vi "Execute.vi"(5 "SleepTerminalArray":refnum<vi>, 6 "ExeRef":refnum<vi>, 7 "ActiveTerminalArray":refnum<vi>, 8 "error in (no error)":errorcluster, 9 "Json_In":string, 10 "VariableRef":T2, 11 "Info":T1) -> (0 "Error Out":errorcluster, 1 "NumResultArray":dbl[](array[numeric]), 2 "StrResultArray":string[](array[string]), 3 "StrResult":string, 4 "NumResult":dbl)   [LabVIEW 2018, in "File.lvlib"]
uses:
  File.lvlib
  <userlib>/_OpenG.lib/dictionary/dictionary.llb/Dictionary Object RefNum__ogtk.ctl
  <userlib>/_OpenG.lib/dictionary/dictionary.llb/Dictionary Object RefNum - Enum__ogtk.ctl
  <userlib>/_MGI/File/MGI Create Directory Chain Behavior Enum.ctl
  <vilib>/addons/_JKI.lib/Serialization/JSON/JKI JSON Serialization.lvlib
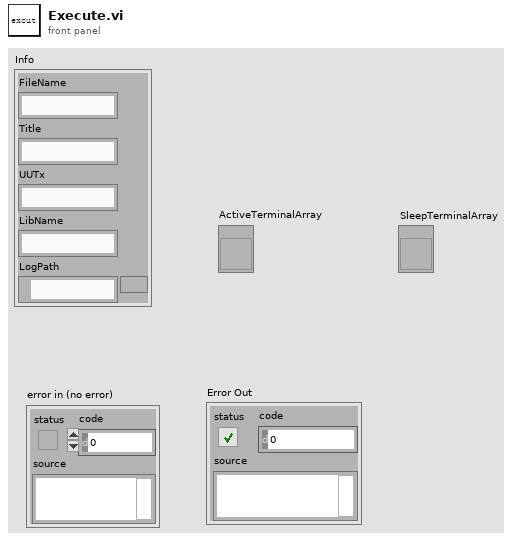
[diagram p1: front panel]
types:
  T1 = cluster{"FileName":string, "Title":string, "UUTx":string, "LibName":string, "LogPath":path}
  T2 = typedef "Dictionary Object RefNum__ogtk.ctl" = refnum<k1>
  T3 = cluster{"SetPath":cluster{"json":cluster{"Method":string, "Path":string, "PathType":string}}, "CreatFile":cluster{"json":cluster{"Method":string, "Path":string, "Operation":string, "Access":string, "DisableBuffering":bool}}, "CreatFolder":cluster{"json":cluster{"Method":string, "Path":string}}, "Delete":cluster{"json":cluster{"Method":string, "Path":string, "EntireHierarchy":bool, "Confirm":bool}}, "ReadTextFile":cluster{"json":cluster{"Method":string, "Path":string, "count":i32}}, "WriteTextFile":cluster{"json":cluster{"Method":string, "Path":string, "Offset":i64, "Position":string, "Text":string}}, "ReadBinFile":cluster{"json":cluster{"Method":string, "Path":string, "Count":i32, "ByteOrder":string}}, "WriteBinFile":cluster{"json":cluster{"Method":string, "Path":string, "ByteOrder":string, "PrependDataSize":bool, "Bin":string}}, "ReadFileMD5":cluster{"json":cluster{"Method":string, "Path":string}}, "Move":cluster{"json":cluster{"Method":string, "Path":string, "TargetPath":string, "Overwrite":bool}}, "Copy":cluster{"json":cluster{"Method":string, "Path":string, "TargetPath":string, "Overwrite":bool}}, "GetFileSize":cluster{"json":cluster{"Method":string, "Path":string}}, "CheckifFileorFolderExists":cluster{"json":cluster{"Method":string, "Path":string}}, "ListFolder":cluster{"json":cluster{"Method":string, "Path":string, "Type":string}}}
  T4 = typedef "MGI Create Directory Chain Behavior Enum.ctl" = enum16{"Auto Detect", "Path Contains a File", "Path Does Not Contain a File"}
  T5 = enum16{"open", "replace", "create", "open or create", "replace or create", "replace or create with confirmation"}
  T6 = enum16{"big-endian, network order", "native, host order", "little-endian"}
  T7 = cluster{"json":cluster{"Method":string, "Path":string, "PathType":string}}
  T8 = enum32{"invalid app kind", "Development System", "Run Time System", "Student Edition", "Embedded LabVIEW", "Evaluation", "Custom"}
  T9 = cluster{"json":cluster{"Method":string, "Path":string, "Operation":string, "Access":string, "DisableBuffering":bool}}
  T10 = cluster{"json":cluster{"Method":string, "Path":string}}
  T11 = cluster{"json":cluster{"Method":string, "Path":string, "EntireHierarchy":bool, "Confirm":bool}}
  T12 = cluster{"json":cluster{"Method":string, "Path":string, "count":i32}}
  T13 = cluster{"json":cluster{"Method":string, "Path":string, "Offset":i64, "Position":string, "Text":string}}
  T14 = cluster{"json":cluster{"Method":string, "Path":string, "Count":i32, "ByteOrder":string}}
  T15 = cluster{"json":cluster{"Method":string, "Path":string, "ByteOrder":string, "PrependDataSize":bool, "Bin":string}}
  T16 = cluster{"json":cluster{"Method":string, "Path":string, "TargetPath":string, "Overwrite":bool}}
  T17 = cluster{"json":cluster{"Method":string, "Path":string, "Type":string}}
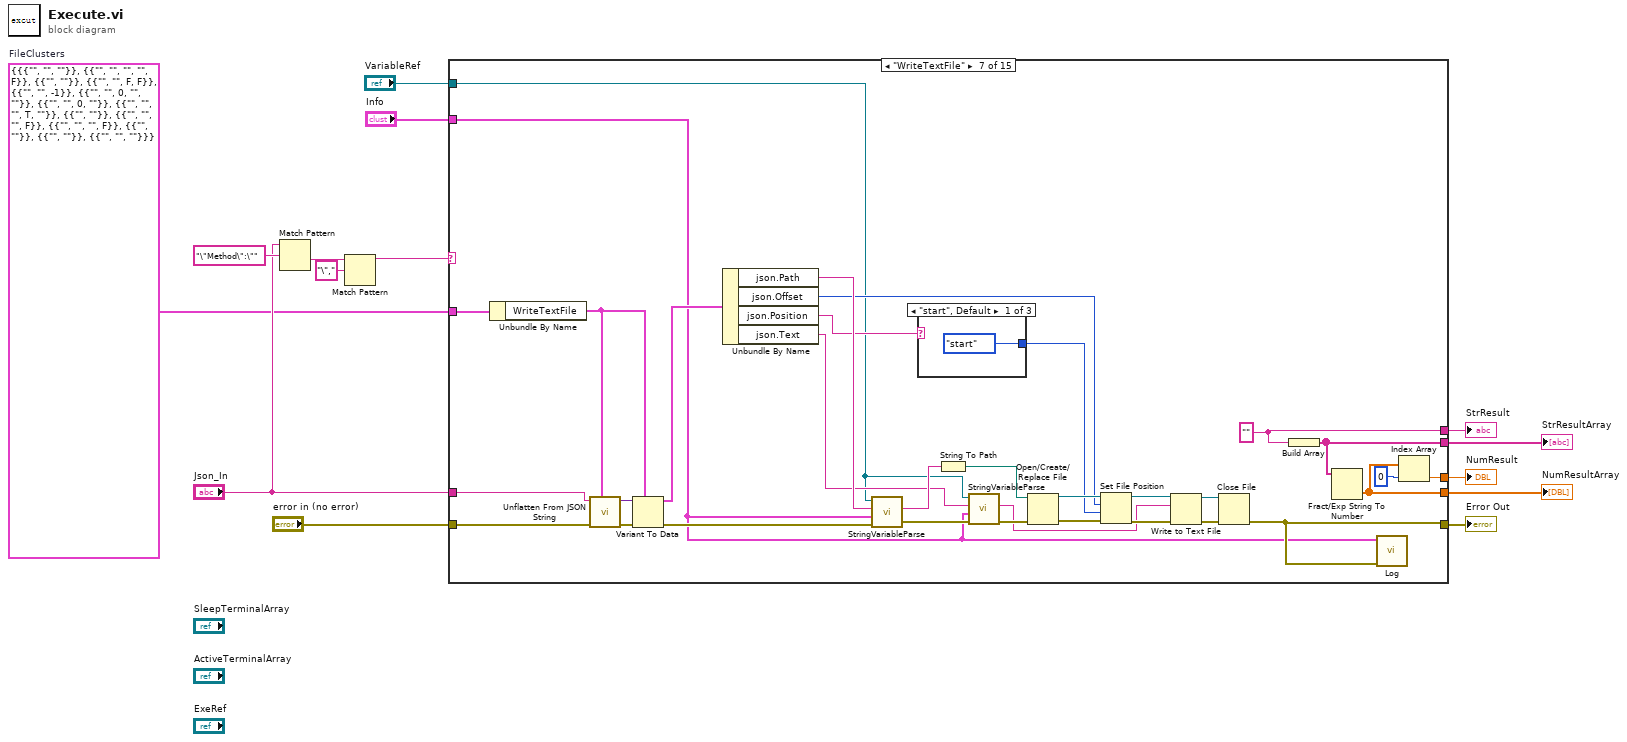
[diagram p0: block diagram]
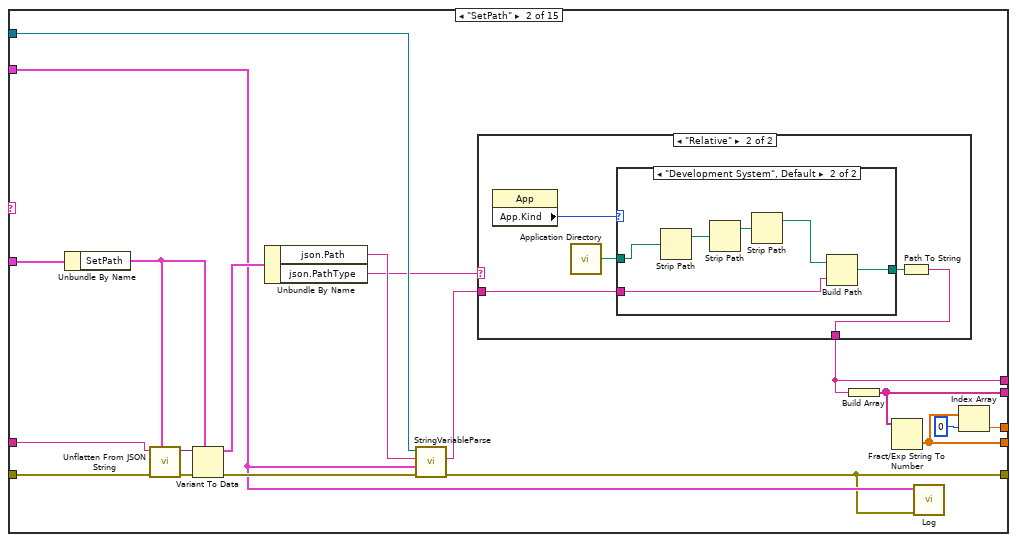
[diagram p3: hidden frame]
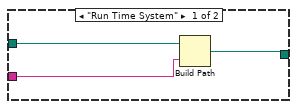
[diagram p5: hidden frame]
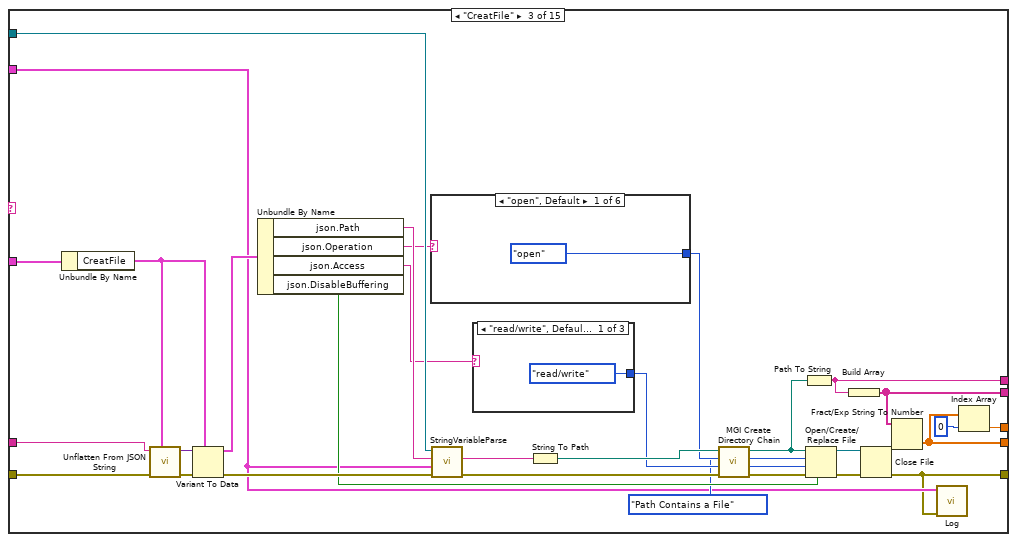
[diagram p6: hidden frame]
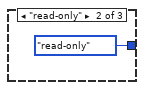
[diagram p7: hidden frame]
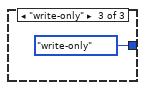
[diagram p8: hidden frame]
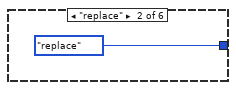
[diagram p9: hidden frame]
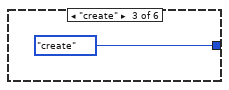
[diagram p10: hidden frame]
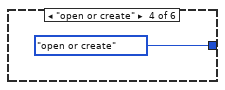
[diagram p11: hidden frame]
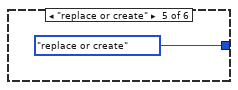
[diagram p12: hidden frame]
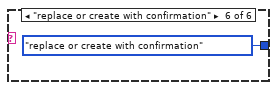
[diagram p13: hidden frame]
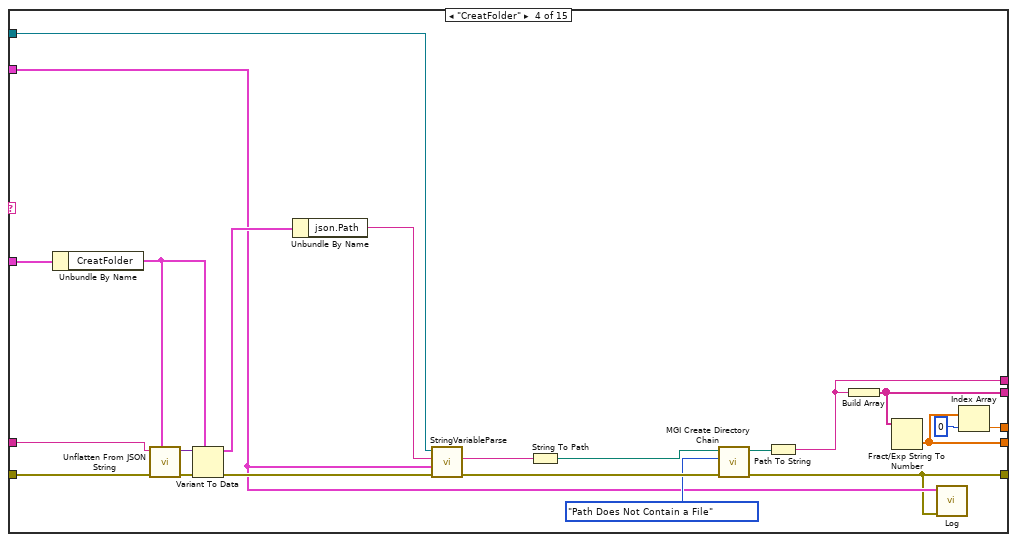
[diagram p14: hidden frame]
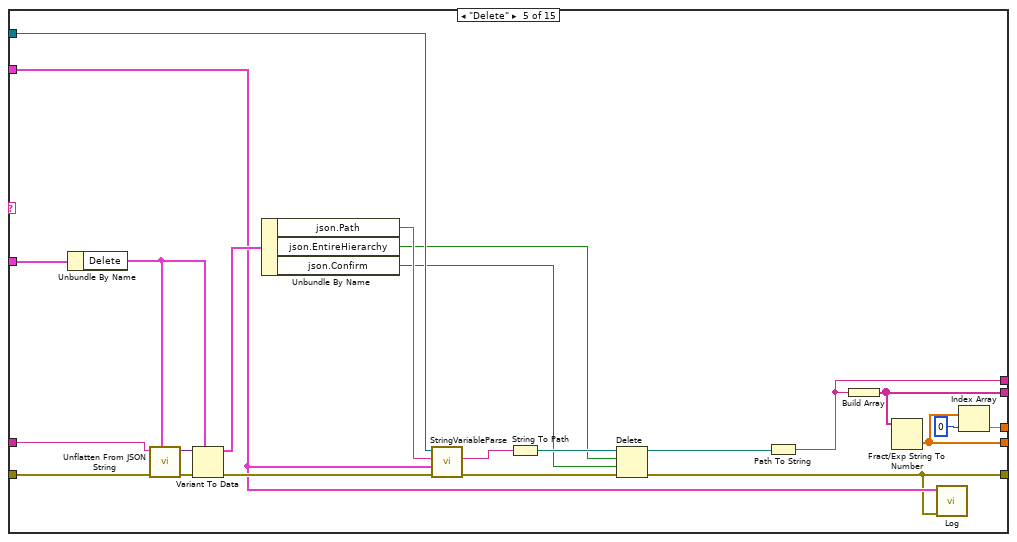
[diagram p15: hidden frame]
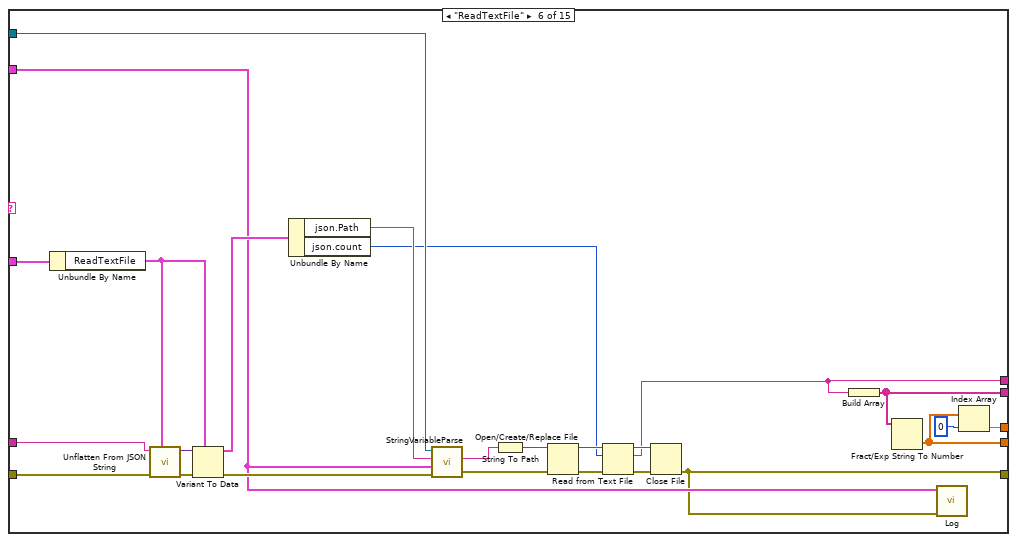
[diagram p16: hidden frame]
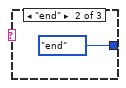
[diagram p17: hidden frame]
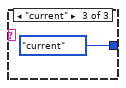
[diagram p18: hidden frame]
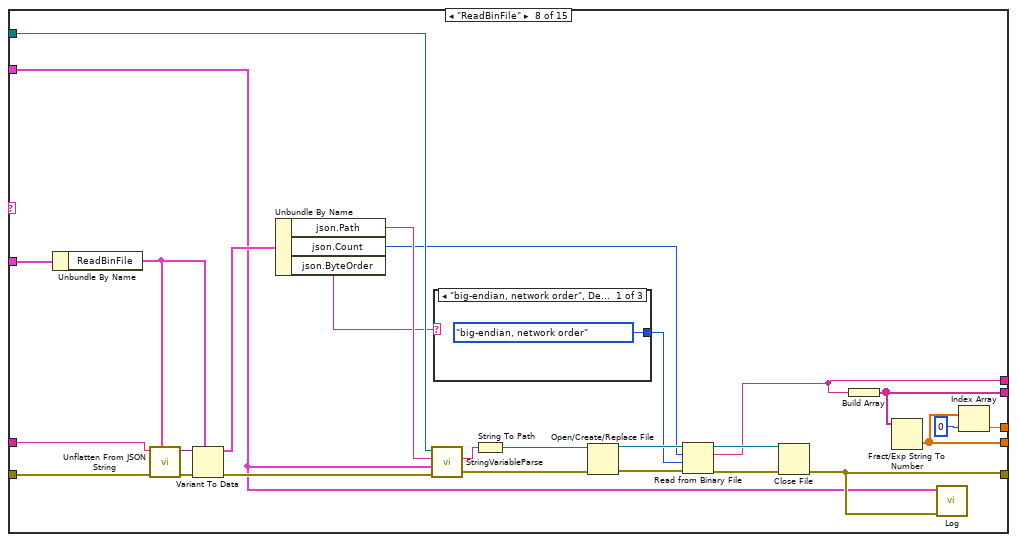
[diagram p19: hidden frame]
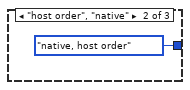
[diagram p20: hidden frame]
diagram:
  w1 = T3 {"SetPath"={"json"={"Method"="", "Path"="", "PathType"=""}}, "CreatFile"={"json"={"Method"="", "Path"="", "Operation"="", "Access"="", "DisableBuffering"=FALSE}}, "CreatFolder"={"json"={"Method"="", "Path"=""}}, "Delete"={"json"={"Method"="", "Path"="", "EntireHierarchy"=FALSE, "Confirm"=FALSE}}, "ReadTextFile"={"json"={"Method"="", "Path"="", "count"=-1}}, "WriteTextFile"={"json"={"Method"="", "Path"="", "Offset"=0, "Position"="", "Text"=""}}, "ReadBinFile"={"json"={"Method"="", "Path"="", "Count"=0, "ByteOrder"=""}}, "WriteBinFile"={"json"={"Method"="", "Path"="", "ByteOrder"="", "PrependDataSize"=TRUE, "Bin"=""}}, "ReadFileMD5"={"json"={"Method"="", "Path"=""}}, "Move"={"json"={"Method"="", "Path"="", "TargetPath"="", "Overwrite"=FALSE}}, "Copy"={"json"={"Method"="", "Path"="", "TargetPath"="", "Overwrite"=FALSE}}, "GetFileSize"={"json"={"Method"="", "Path"=""}}, "CheckifFileorFolderExists"={"json"={"Method"="", "Path"=""}}, "ListFolder"={"json"={"Method"="", "Path"="", "Type"=""}}}  # FileClusters
  n1 = Match Pattern(string="Json_In", regular expression="\"Method\":\"") -> (after substring=w4:string)  [unwired: 1 in, 3 out]
  n2 = Match Pattern(string=w4, regular expression="\",") -> (before substring=w2:string)  [unwired: 1 in, 3 out]
  n3 = case shown="\"WriteTextFile\"" w2 {
    tunnel: "Json_In" -> [_ w31 w76 w107 w130 w155 w187 w217 w248 w271 w296 w321 w342 w365 w388]
    tunnel: [w15 w16 w50 w89 w111 w139 w174 w206 w237 w255 w276 w301 w327 w350 w374] -> w14
    tunnel: "error in (no error)" -> [w15 w30 w75 w106 w129 w154 w186 w216 w247 w270 w295 w320 w341 w364 w387]
    tunnel: [_ w18 w52 w91 w118 w134 w159 w194 w224 w256 w275 w300 w325 w348 w370] -> w12
    tunnel: "VariableRef" -> [_ w23 w68 w99 w122 w147 w162 w204 w235 w260 w284 w309 w331 w354 w378]
    tunnel: [_ w24 w69 w100 w123 w148 w180 w210 w241 w264 w289 w314 w335 w358 w369] -> w11
    tunnel: [_ w27 w72 w103 w126 w151 w183 w213 w244 w267 w292 w317 w338 w361 w384] -> w10
    tunnel: [_ w29 w74 w105 w128 w153 w185 w215 w246 w269 w294 w319 w340 w363 w386] -> w9
    tunnel: "Info" -> [_ w17 w51 w90 w117 w143 w161 w203 w234 w259 w282 w307 w330 w353 w377]
    tunnel: w1 -> [_ w26 w71 w102 w125 w150 w182 w212 w243 w266 w291 w316 w337 w360 w383]
    frame Default {
    }
    frame "SetPath" {
      n4 = Unbundle By Name(w26) -> ("SetPath"=w25:T7)
      n5 = call <vilib>:"Unflatten From JSON String.vi"("Type and Defaults"=w25, "error in (no error)"=w30, "JSON String"=w31) -> ("error out"=w33:errorcluster, "Variant"=w34:variant)  [unwired: 7 in]
      n6 = Variant To Data(error in=w33, type=w25, Variant=w34) -> (data=w32:T7, error out=w21:errorcluster)
      n7 = Unbundle By Name(w32) -> ("json.Path"=w22:string, "json.PathType"=w20:string)
      n8 = call "StringVariableParse.vi"("error in"=w21, "Info"=w17, "in"=w22, "dictionary"=w23) -> ("error out"=w16:errorcluster, "out"=w19:string)  [unwired: 5 in, 1 out]
      n9 = case shown="\"Relative\"" w20 {
        tunnel: w19 -> [w35 w38]
        tunnel: [w35 w36] -> w18
        frame "Absolute", Default {
        }
        frame "Relative" {
          n10 = property class="App"() -> ("App.Kind"=w39:T8)  [unwired: 2 in, 2 out]
          n11 = call <vilib>:"Application Directory.vi"() -> ("Application Directory"=w40:path)
          n12 = case shown="\"Development System\", Default" w39 {
            tunnel: [w43 w47] -> w37
            tunnel: w40 -> [w42 w45]
            tunnel: w38 -> [w41 w44]
            frame "Run Time System" {
              n13 = Build Path(base path=w42, name or relative path=w41) -> (appended path=w43:path)
            }
            frame "Development System", Default {
              n14 = Strip Path(path=w45) -> (stripped path=w49:path)  [unwired: 1 out]
              n15 = Strip Path(path=w49) -> (stripped path=w48:path)  [unwired: 1 out]
              n16 = Strip Path(path=w48) -> (stripped path=w46:path)  [unwired: 1 out]
              n17 = Build Path(base path=w46, name or relative path=w44) -> (appended path=w47:path)
            }
          }
          n18 = Path To String(path=w37) -> (string=w36:string)
        }
      }
      n19 = Build Array(w18) -> (w24:string[])
      n20 = Fract/Exp String To Number(string=w24) -> (number=w29:dbl[])  [unwired: 3 in, 1 out]
      n21 = call "Log.vi"("error in"=w16, "Info"=w17) -> ()  [unwired: 10 in]
      n22 = Index Array(array=w29, index=0) -> (element=w27:dbl)
    }
    frame "CreatFile" {
      n23 = Unbundle By Name(w71) -> ("CreatFile"=w70:T9)
      n24 = call <vilib>:"Unflatten From JSON String.vi"("Type and Defaults"=w70, "error in (no error)"=w75, "JSON String"=w76) -> ("error out"=w78:errorcluster, "Variant"=w79:variant)  [unwired: 7 in]
      n25 = Variant To Data(error in=w78, type=w70, Variant=w79) -> (data=w77:T9, error out=w66:errorcluster)
      n26 = Unbundle By Name(w77) -> ("json.Path"=w67:string, "json.Operation"=w62:string, "json.Access"=w60:string, "json.DisableBuffering"=w59:bool)
      n27 = case shown="\"open\", Default" w62 {
        tunnel: [T5."open" ("operation (0:open)") T5."replace" ("operation (0:open)") T5."create" ("operation (0:open)") T5."open or create" ("operation (0:open)") T5."replace or create" ("operation (0:open)") T5."replace or create with confirmation" ("operation (0:open)")] -> w63
        frame "open", Default {
        }
        frame "replace" {
        }
        frame "create" {
        }
        frame "open or create" {
        }
        frame "replace or create" {
        }
        frame "replace or create with confirmation" {
        }
      }
      n28 = call "StringVariableParse.vi"("error in"=w66, "Info"=w51, "in"=w67, "dictionary"=w68) -> ("error out"=w58:errorcluster, "out"=w65:string)  [unwired: 5 in, 1 out]
      n29 = case shown="\"read/write\", Default" w60 {
        tunnel: [enum16{"read/write", "read-only", "write-only"}."read/write" ("access (0:read/write)") enum16{"read/write", "read-only", "write-only"}."read-only" ("access (0:read/write)") enum16{"read/write", "read-only", "write-only"}."write-only" ("access (0:read/write)")] -> w61
        frame "read/write", Default {
        }
        frame "read-only" {
        }
        frame "write-only" {
        }
      }
      n30 = String To Path(string=w65) -> (path=w64:path)
      n31 = call <userlib>:"MGI Create Directory Chain.vi"("Error In"=w58, "File Presence (Auto Detect)"=MGI_Create_Directory_Chain_Behavior_Enum."Path Contains a File", "Path"=w64) -> ("Error Out"=w57:errorcluster, "Duplicate Path"=w53:path)  [unwired: 7 in]
      n32 = Path To String(path=w53) -> (string=w52:string)
      n33 = Open/Create/Replace File(file path (use dialog)=w53, error in=w57, operation (0:open)=w63, access (0:read/write)=w61, disable buffering (F)=w59) -> (refnum out=w55:refnum<file>, error out=w54:errorcluster)  [unwired: 1 in, 1 out]
      n34 = Build Array(w52) -> (w69:string[])
      n35 = Close File(refnum=w55, error in=w54) -> (error out=w50:errorcluster)  [unwired: 1 out]
      n36 = Fract/Exp String To Number(string=w69) -> (number=w74:dbl[])  [unwired: 3 in, 1 out]
      n37 = call "Log.vi"("error in"=w50, "Info"=w51) -> ()  [unwired: 10 in]
      n38 = Index Array(array=w74, index=0) -> (element=w72:dbl)
    }
    frame "CreatFolder" {
      n39 = Unbundle By Name(w102) -> ("CreatFolder"=w101:T10)
      n40 = call <vilib>:"Unflatten From JSON String.vi"("Type and Defaults"=w101, "error in (no error)"=w106, "JSON String"=w107) -> ("error out"=w109:errorcluster, "Variant"=w110:variant)  [unwired: 7 in]
      n41 = Variant To Data(error in=w109, type=w101, Variant=w110) -> (data=w108:T10, error out=w97:errorcluster)
      n42 = Unbundle By Name(w108) -> ("json.Path"=w98:string)
      n43 = call "StringVariableParse.vi"("error in"=w97, "Info"=w90, "in"=w98, "dictionary"=w99) -> ("error out"=w94:errorcluster, "out"=w96:string)  [unwired: 5 in, 1 out]
      n44 = String To Path(string=w96) -> (path=w95:path)
      n45 = call <userlib>:"MGI Create Directory Chain.vi"("Error In"=w94, "File Presence (Auto Detect)"=MGI_Create_Directory_Chain_Behavior_Enum."Path Does Not Contain a File", "Path"=w95) -> ("Error Out"=w89:errorcluster, "Duplicate Path"=w92:path)  [unwired: 7 in]
      n46 = Path To String(path=w92) -> (string=w91:string)
      n47 = Build Array(w91) -> (w100:string[])
      n48 = Fract/Exp String To Number(string=w100) -> (number=w105:dbl[])  [unwired: 3 in, 1 out]
      n49 = call "Log.vi"("error in"=w89, "Info"=w90) -> ()  [unwired: 10 in]
      n50 = Index Array(array=w105, index=0) -> (element=w103:dbl)
    }
    frame "Delete" {
      n51 = Unbundle By Name(w125) -> ("Delete"=w124:T11)
      n52 = call <vilib>:"Unflatten From JSON String.vi"("Type and Defaults"=w124, "error in (no error)"=w129, "JSON String"=w130) -> ("error out"=w132:errorcluster, "Variant"=w133:variant)  [unwired: 7 in]
      n53 = Variant To Data(error in=w132, type=w124, Variant=w133) -> (data=w131:T11, error out=w120:errorcluster)
      n54 = Unbundle By Name(w131) -> ("json.Path"=w121:string, "json.EntireHierarchy"=w115:bool, "json.Confirm"=w114:bool)
      n55 = call "StringVariableParse.vi"("error in"=w120, "Info"=w117, "in"=w121, "dictionary"=w122) -> ("error out"=w113:errorcluster, "out"=w119:string)  [unwired: 5 in, 1 out]
      n56 = String To Path(string=w119) -> (path=w116:path)
      n57 = Delete(path (use dialog)=w116, entire hierarchy (F)=w115, confirm (F)=w114, error in=w113) -> (deleted path=w112:path, error out=w111:errorcluster)  [unwired: 1 in, 1 out]
      n58 = Path To String(path=w112) -> (string=w118:string)
      n59 = Build Array(w118) -> (w123:string[])
      n60 = Fract/Exp String To Number(string=w123) -> (number=w128:dbl[])  [unwired: 3 in, 1 out]
      n61 = call "Log.vi"("error in"=w111, "Info"=w117) -> ()  [unwired: 10 in]
      n62 = Index Array(array=w128, index=0) -> (element=w126:dbl)
    }
    frame "ReadTextFile" {
      n63 = Unbundle By Name(w150) -> ("ReadTextFile"=w149:T12)
      n64 = call <vilib>:"Unflatten From JSON String.vi"("Type and Defaults"=w149, "error in (no error)"=w154, "JSON String"=w155) -> ("error out"=w157:errorcluster, "Variant"=w158:variant)  [unwired: 7 in]
      n65 = Variant To Data(error in=w157, type=w149, Variant=w158) -> (data=w156:T12, error out=w145:errorcluster)
      n66 = Unbundle By Name(w156) -> ("json.Path"=w146:string, "json.count"=w137:i32)
      n67 = call "StringVariableParse.vi"("error in"=w145, "Info"=w143, "in"=w146, "dictionary"=w147) -> ("error out"=w135:errorcluster, "out"=w144:string)  [unwired: 5 in, 1 out]
      n68 = String To Path(string=w144) -> (path=w136:path)
      n69 = Open/Create/Replace File(file path (use dialog)=w136, error in=w135) -> (refnum out=w138:refnum<file>, error out=w142:errorcluster)  [unwired: 4 in, 1 out]
      n70 = Read from Text File(file (use dialog)=w138, count=w137, error in=w142) -> (refnum out=w140:refnum<file>, text=w134:string, error out=w141:errorcluster)  [unwired: 1 in, 1 out]
      n71 = Close File(refnum=w140, error in=w141) -> (error out=w139:errorcluster)  [unwired: 1 out]
      n72 = Build Array(w134) -> (w148:string[])
      n73 = Fract/Exp String To Number(string=w148) -> (number=w153:dbl[])  [unwired: 3 in, 1 out]
      n74 = call "Log.vi"("error in"=w139, "Info"=w143) -> ()  [unwired: 10 in]
      n75 = Index Array(array=w153, index=0) -> (element=w151:dbl)
    }
    frame "WriteTextFile" {
      w159 = ""
      n76 = Unbundle By Name(w182) -> ("WriteTextFile"=w181:T13)
      n77 = call <vilib>:"Unflatten From JSON String.vi"("Type and Defaults"=w181, "error in (no error)"=w186, "JSON String"=w187) -> ("error out"=w189:errorcluster, "Variant"=w190:variant)  [unwired: 7 in]
      n78 = Variant To Data(error in=w189, type=w181, Variant=w190) -> (data=w188:T13, error out=w178:errorcluster)
      n79 = Unbundle By Name(w188) -> ("json.Path"=w179:string, "json.Offset"=w168:i64, "json.Position"=w166:string, "json.Text"=w163:string)
      n80 = call "StringVariableParse.vi"("error in"=w178, "Info"=w161, "in"=w179, "dictionary"=w162) -> ("error out"=w165:errorcluster, "out"=w177:string)  [unwired: 5 in, 1 out]
      n81 = case shown="\"start\", Default" w166 {
        tunnel: [enum16{"start", "end", "current"}."start" ("from (0:start)") enum16{"start", "end", "current"}."end" ("from (0:start)") enum16{"start", "end", "current"}."current" ("from (0:start)")] -> w167
        frame "start", Default {
        }
        frame "end" {
        }
        frame "current" {
        }
      }
      n82 = String To Path(string=w177) -> (path=w173:path)
      n83 = call "StringVariableParse.vi"("error in"=w165, "Info"=w161, "in"=w163, "dictionary"=w162) -> ("error out"=w164:errorcluster, "out"=w160:string)  [unwired: 5 in, 1 out]
      n84 = Open/Create/Replace File(file path (use dialog)=w173, error in=w164) -> (refnum out=w172:refnum<file>, error out=w169:errorcluster)  [unwired: 4 in, 1 out]
      n85 = Set File Position(offset (in bytes) (0)=w168, refnum=w172, from (0:start)=w167, error in=w169) -> (refnum out=w171:refnum<file>, error out=w170:errorcluster)
      n86 = Write to Text File(file (use dialog)=w171, text=w160, error in=w170) -> (refnum out=w175:refnum<file>, error out=w176:errorcluster)  [unwired: 1 in, 1 out]
      n87 = Close File(refnum=w175, error in=w176) -> (error out=w174:errorcluster)  [unwired: 1 out]
      n88 = Build Array(w159) -> (w180:string[])
      n89 = Fract/Exp String To Number(string=w180) -> (number=w185:dbl[])  [unwired: 3 in, 1 out]
      n90 = call "Log.vi"("error in"=w174, "Info"=w161) -> ()  [unwired: 10 in]
      n91 = Index Array(array=w185, index=0) -> (element=w183:dbl)
    }
    frame "ReadBinFile" {
      n92 = Unbundle By Name(w212) -> ("ReadBinFile"=w211:T14)
      n93 = call <vilib>:"Unflatten From JSON String.vi"("Type and Defaults"=w211, "error in (no error)"=w216, "JSON String"=w217) -> ("error out"=w219:errorcluster, "Variant"=w220:variant)  [unwired: 7 in]
      n94 = Variant To Data(error in=w219, type=w211, Variant=w220) -> (data=w218:T14, error out=w208:errorcluster)
      n95 = Unbundle By Name(w218) -> ("json.Path"=w209:string, "json.Count"=w197:i32, "json.ByteOrder"=w195:string)
      n96 = call "StringVariableParse.vi"("error in"=w208, "Info"=w203, "in"=w209, "dictionary"=w204) -> ("error out"=w202:errorcluster, "out"=w207:string)  [unwired: 5 in, 1 out]
      n97 = case shown="\"big-endian, network order\", Default" w195 {
        tunnel: [T6."big-endian, network order" ("byte order (0:big-endian, network order)") T6."native, host order" ("byte order (0:big-endian, network order)") T6."native, host order" ("byte order (0:big-endian, network order)")] -> w196
        frame "big-endian, network order", Default {
        }
        frame "host order", "native" {
        }
        frame "little-endian" {
        }
      }
      n98 = String To Path(string=w207) -> (path=w205:path)
      n99 = Open/Create/Replace File(file path (use dialog)=w205, error in=w202) -> (refnum out=w201:refnum<file>, error out=w200:errorcluster)  [unwired: 4 in, 1 out]
      n100 = Read from Binary File(8:w200, 9:w196, 10:w197, 11:w201) -> (0:w198:errorcluster, 2:w194:string, 3:w199:refnum<file>)  [unwired: 2 in, 1 out]
      n101 = Close File(refnum=w199, error in=w198) -> (error out=w206:errorcluster)  [unwired: 1 out]
      n102 = Build Array(w194) -> (w210:string[])
      n103 = Fract/Exp String To Number(string=w210) -> (number=w215:dbl[])  [unwired: 3 in, 1 out]
      n104 = call "Log.vi"("error in"=w206, "Info"=w203) -> ()  [unwired: 10 in]
      n105 = Index Array(array=w215, index=0) -> (element=w213:dbl)
    }
    frame "WriteBinFile" {
      w224 = ""
      n106 = Unbundle By Name(w243) -> ("WriteBinFile"=w242:T15)
      n107 = call <vilib>:"Unflatten From JSON String.vi"("Type and Defaults"=w242, "error in (no error)"=w247, "JSON String"=w248) -> ("error out"=w250:errorcluster, "Variant"=w251:variant)  [unwired: 7 in]
      n108 = Variant To Data(error in=w250, type=w242, Variant=w251) -> (data=w249:T15, error out=w239:errorcluster)
      n109 = Unbundle By Name(w249) -> ("json.Path"=w240:string, "json.ByteOrder"=w227:string, "json.PrependDataSize"=w225:bool, "json.Bin"=w226:string)
      n110 = call "StringVariableParse.vi"("error in"=w239, "Info"=w234, "in"=w240, "dictionary"=w235) -> ("error out"=w233:errorcluster, "out"=w238:string)  [unwired: 5 in, 1 out]
      n111 = case shown="\"big-endian, network order\", Default" w227 {
        tunnel: [T6."big-endian, network order" ("byte order (0:big-endian, network order)") T6."native, host order" ("byte order (0:big-endian, network order)") T6."native, host order" ("byte order (0:big-endian, network order)")] -> w228
        frame "big-endian, network order", Default {
        }
        frame "host order", "native" {
        }
        frame "little-endian" {
        }
      }
      n112 = String To Path(string=w238) -> (path=w236:path)
      n113 = Open/Create/Replace File(file path (use dialog)=w236, error in=w233) -> (refnum out=w232:refnum<file>, error out=w231:errorcluster)  [unwired: 4 in, 1 out]
      n114 = Write to Binary File(file (use dialog)=w232, data=w226, error in=w231, 5:w225, 9:w228) -> (refnum out=w230:refnum<file>, error out=w229:errorcluster)  [unwired: 1 in, 1 out]
      n115 = Close File(refnum=w230, error in=w229) -> (error out=w237:errorcluster)  [unwired: 1 out]
      n116 = Build Array(w224) -> (w241:string[])
      n117 = Fract/Exp String To Number(string=w241) -> (number=w246:dbl[])  [unwired: 3 in, 1 out]
      n118 = call "Log.vi"("error in"=w237, "Info"=w234) -> ()  [unwired: 10 in]
      n119 = Index Array(array=w246, index=0) -> (element=w244:dbl)
    }
    frame "ReadFileMD5" {
      n120 = Unbundle By Name(w266) -> ("ReadFileMD5"=w265:T10)
      n121 = call <vilib>:"Unflatten From JSON String.vi"("Type and Defaults"=w265, "error in (no error)"=w270, "JSON String"=w271) -> ("error out"=w273:errorcluster, "Variant"=w274:variant)  [unwired: 7 in]
      n122 = Variant To Data(error in=w273, type=w265, Variant=w274) -> (data=w272:T10, error out=w262:errorcluster)
      n123 = Unbundle By Name(w272) -> ("json.Path"=w263:string)
      n124 = call "StringVariableParse.vi"("error in"=w262, "Info"=w259, "in"=w263, "dictionary"=w260) -> ("error out"=w258:errorcluster, "out"=w261:string)  [unwired: 5 in, 1 out]
      n125 = String To Path(string=w261) -> (path=w257:path)
      n126 = call <vilib>:"MD5Checksum File.vi"("error in (no error)"=w258, "Path"=w257) -> ("error out"=w255:errorcluster, "MD5 message-digest"=w256:string)  [unwired: 8 in]
      n127 = Build Array(w256) -> (w264:string[])
      n128 = Fract/Exp String To Number(string=w264) -> (number=w269:dbl[])  [unwired: 3 in, 1 out]
      n129 = call "Log.vi"("error in"=w255, "Info"=w259) -> ()  [unwired: 10 in]
      n130 = Index Array(array=w269, index=0) -> (element=w267:dbl)
    }
    frame "Move" {
      w275 = ""
      n131 = Unbundle By Name(w291) -> ("Move"=w290:T16)
      n132 = call <vilib>:"Unflatten From JSON String.vi"("Type and Defaults"=w290, "error in (no error)"=w295, "JSON String"=w296) -> ("error out"=w298:errorcluster, "Variant"=w299:variant)  [unwired: 7 in]
      n133 = Variant To Data(error in=w298, type=w290, Variant=w299) -> (data=w297:T16, error out=w287:errorcluster)
      n134 = Unbundle By Name(w297) -> ("json.Path"=w288:string, "json.TargetPath"=w283:string, "json.Overwrite"=w278:bool)
      n135 = call "StringVariableParse.vi"("error in"=w287, "Info"=w282, "in"=w288, "dictionary"=w284) -> ("error out"=w285:errorcluster, "out"=w286:string)  [unwired: 5 in, 1 out]
      n136 = String To Path(string=w286) -> (path=w280:path)
      n137 = call "StringVariableParse.vi"("error in"=w285, "Info"=w282, "in"=w283, "dictionary"=w284) -> ("error out"=w277:errorcluster, "out"=w281:string)  [unwired: 5 in, 1 out]
      n138 = String To Path(string=w281) -> (path=w279:path)
      n139 = Move(source path=w280, error in=w277, 9:w278, 10:w279) -> (error out=w276:errorcluster)  [unwired: 1 in, 2 out]
      n140 = Build Array(w275) -> (w289:string[])
      n141 = Fract/Exp String To Number(string=w289) -> (number=w294:dbl[])  [unwired: 3 in, 1 out]
      n142 = call "Log.vi"("error in"=w276, "Info"=w282) -> ()  [unwired: 10 in]
      n143 = Index Array(array=w294, index=0) -> (element=w292:dbl)
    }
    frame "Copy" {
      w300 = ""
      n144 = Unbundle By Name(w316) -> ("Copy"=w315:T16)
      n145 = call <vilib>:"Unflatten From JSON String.vi"("Type and Defaults"=w315, "error in (no error)"=w320, "JSON String"=w321) -> ("error out"=w323:errorcluster, "Variant"=w324:variant)  [unwired: 7 in]
      n146 = Variant To Data(error in=w323, type=w315, Variant=w324) -> (data=w322:T16, error out=w312:errorcluster)
      n147 = Unbundle By Name(w322) -> ("json.Path"=w313:string, "json.TargetPath"=w308:string, "json.Overwrite"=w303:bool)
      n148 = call "StringVariableParse.vi"("error in"=w312, "Info"=w307, "in"=w313, "dictionary"=w309) -> ("error out"=w310:errorcluster, "out"=w311:string)  [unwired: 5 in, 1 out]
      n149 = String To Path(string=w311) -> (path=w305:path)
      n150 = call "StringVariableParse.vi"("error in"=w310, "Info"=w307, "in"=w308, "dictionary"=w309) -> ("error out"=w302:errorcluster, "out"=w306:string)  [unwired: 5 in, 1 out]
      n151 = String To Path(string=w306) -> (path=w304:path)
      n152 = Copy(8:w302, 9:w303, 10:w304, 11:w305) -> (0:w301:errorcluster)  [unwired: 1 in, 2 out]
      n153 = Build Array(w300) -> (w314:string[])
      n154 = Fract/Exp String To Number(string=w314) -> (number=w319:dbl[])  [unwired: 3 in, 1 out]
      n155 = call "Log.vi"("error in"=w301, "Info"=w307) -> ()  [unwired: 10 in]
      n156 = Index Array(array=w319, index=0) -> (element=w317:dbl)
    }
    frame "GetFileSize" {
      n157 = Unbundle By Name(w337) -> ("GetFileSize"=w336:T10)
      n158 = call <vilib>:"Unflatten From JSON String.vi"("Type and Defaults"=w336, "error in (no error)"=w341, "JSON String"=w342) -> ("error out"=w344:errorcluster, "Variant"=w345:variant)  [unwired: 7 in]
      n159 = Variant To Data(error in=w344, type=w336, Variant=w345) -> (data=w343:T10, error out=w333:errorcluster)
      n160 = Unbundle By Name(w343) -> ("json.Path"=w334:string)
      n161 = call "StringVariableParse.vi"("error in"=w333, "Info"=w330, "in"=w334, "dictionary"=w331) -> ("error out"=w328:errorcluster, "out"=w332:string)  [unwired: 5 in, 1 out]
      n162 = String To Path(string=w332) -> (path=w329:path)
      n163 = Get File Size(file=w329, error in=w328) -> (size (in bytes)=w326:i64, 0:w327:errorcluster)  [unwired: 1 out]
      n164 = Number To Decimal String(number=w326) -> (decimal integer string=w325:string)  [unwired: 1 in]
      n165 = Build Array(w325) -> (w335:string[])
      n166 = Fract/Exp String To Number(string=w335) -> (number=w340:dbl[])  [unwired: 3 in, 1 out]
      n167 = call "Log.vi"("error in"=w327, "Info"=w330) -> ()  [unwired: 10 in]
      n168 = Index Array(array=w340, index=0) -> (element=w338:dbl)
    }
    frame "CheckifFileorFolderExists" {
      n169 = Unbundle By Name(w360) -> ("CheckifFileorFolderExists"=w359:T10)
      n170 = call <vilib>:"Unflatten From JSON String.vi"("Type and Defaults"=w359, "error in (no error)"=w364, "JSON String"=w365) -> ("error out"=w367:errorcluster, "Variant"=w368:variant)  [unwired: 7 in]
      n171 = Variant To Data(error in=w367, type=w359, Variant=w368) -> (data=w366:T10, error out=w356:errorcluster)
      n172 = Unbundle By Name(w366) -> ("json.Path"=w357:string)
      n173 = call "StringVariableParse.vi"("error in"=w356, "Info"=w353, "in"=w357, "dictionary"=w354) -> ("error out"=w351:errorcluster, "out"=w355:string)  [unwired: 5 in, 1 out]
      n174 = String To Path(string=w355) -> (path=w352:path)
      n175 = call <vilib>:"Check if File or Folder Exists.vi"("error in (no error)"=w351, "path"=w352) -> ("error out"=w350:errorcluster, "file or folder exists?"=w349:bool)  [unwired: 7 in, 1 out]
      n176 = Select(t="True", s=w349, f="False") -> (s? t:f=w348:string)
      n177 = Build Array(w348) -> (w358:string[])
      n178 = Fract/Exp String To Number(string=w358) -> (number=w363:dbl[])  [unwired: 3 in, 1 out]
      n179 = call "Log.vi"("error in"=w350, "Info"=w353) -> ()  [unwired: 10 in]
      n180 = Index Array(array=w363, index=0) -> (element=w361:dbl)
    }
    frame "ListFolder" {
      n181 = Unbundle By Name(w383) -> ("ListFolder"=w382:T17)
      n182 = call <vilib>:"Unflatten From JSON String.vi"("Type and Defaults"=w382, "error in (no error)"=w387, "JSON String"=w388) -> ("error out"=w390:errorcluster, "Variant"=w391:variant)  [unwired: 7 in]
      n183 = Variant To Data(error in=w390, type=w382, Variant=w391) -> (data=w389:T17, error out=w380:errorcluster)
      n184 = Unbundle By Name(w389) -> ("json.Path"=w381:string, "json.Type"=w373:string)
      n185 = call "StringVariableParse.vi"("error in"=w380, "Info"=w377, "in"=w381, "dictionary"=w378) -> ("error out"=w375:errorcluster, "out"=w379:string)  [unwired: 5 in, 1 out]
      n186 = String To Path(string=w379) -> (path=w376:path)
      n187 = List Folder(path=w376, error in=w375) -> (filenames=w371:string[], folder names=w372:string[], error out=w374:errorcluster)  [unwired: 2 in, 1 out]
      n188 = case shown="\"Folder\", Default" w373 {
        tunnel: [w392 w393] -> w369
        tunnel: w372 -> [w392 _]
        tunnel: w371 -> [_ w393]
        frame "Folder", Default {
        }
        frame "File" {
        }
      }
      n189 = Index Array(array=w369) -> (element=w370:string)  [unwired: 1 in]
      n190 = Fract/Exp String To Number(string=w369) -> (number=w386:dbl[])  [unwired: 3 in, 1 out]
      n191 = call "Log.vi"("error in"=w374, "Info"=w377) -> ()  [unwired: 10 in]
      n192 = Index Array(array=w386, index=0) -> (element=w384:dbl)
    }
  }
  "StrResult" <- w12
  "Error Out" <- w14
  "StrResultArray" <- w11
  "NumResult" <- w10
  "NumResultArray" <- w9
